vi "delete vi from lib.vi"(8 "error in":errorcluster, 9 "delete on disk (t)":bool=TRUE, 10 "relative path":string, 11 "Project in":refnum<vi>) -> (0 "error out":errorcluster, 3 "Project out":refnum<vi>, 5 "lib path":path)   [LabVIEW 2013, in "FixedChannelTBModuleDecideFeatures.lvclass"]
uses:
  FixedChannelTBModuleDecideFeatures.lvclass
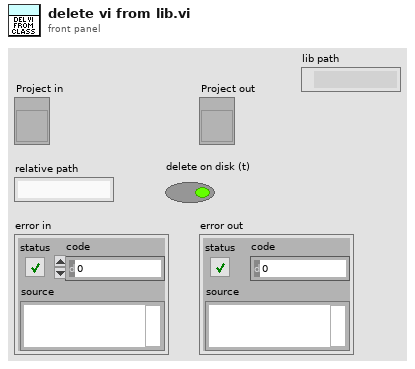
[diagram p1: front panel]
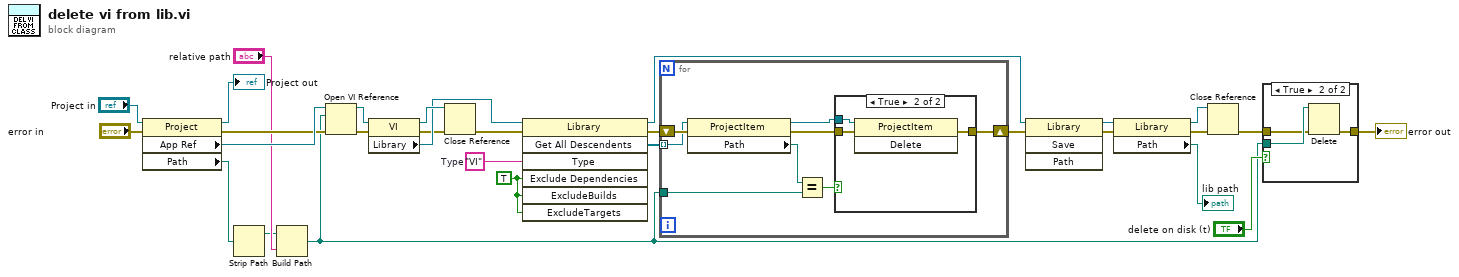
[diagram p0: block diagram]
diagram:
  w18 = TRUE
  w19 = "VI"  # Type
  n1 = property class="Project"(reference="Project in", error in="error in") -> (reference out=→"Project out":refnum<vi>, error out=w14:errorcluster, "App Ref"=w15:refnum<vi>, "Path"=w11:path)
  n2 = Strip Path(path=w11) -> (stripped path=w12:path)  [unwired: 1 out]
  n3 = Build Path(base path=w12, name or relative path="relative path") -> (appended path=w7:path)
  n4 = Open VI Reference(application reference (local)=w15, vi path=w7, error in (no error)=w14) -> (vi reference=w16:refnum<vi>, error out=w17:errorcluster)  [unwired: 3 in]
  n5 = property class="VI"(reference=w16, error in=w17) -> (reference out=w28:refnum<vi>, error out=w20:errorcluster, "Library"=w21:refnum<vi>)
  n6 = Close Reference(reference=w28, error in (no error)=w20) -> (error out=w27:errorcluster)
  n7 = invoke class="Library" method="Get All Descendents"(reference=w21, error in=w27, "Type"=w19, "Exclude Dependencies"=w18, "ExcludeBuilds"=w18, "ExcludeTargets"=w18) -> (reference out=w26:refnum<vi>, error out=w23:errorcluster, "All Descendents"=w22:refnum<vi>[])  [unwired: 1 in, 4 out]
  n8 = for {
    tunnel: w22 -> [w36] mode=indexing
    shift-right: [w30] -> w24
    shift-left: w23 -> [w37]
    tunnel: w7 -> [w34]
    n9 = property class="ProjectItem"(reference=w36, error in=w37) -> (reference out=w31:refnum<vi>, error out=w32:errorcluster, "Path"=w35:path)
    n10 = Equal?(x=w35, y=w34) -> (x = y?=w33:bool)
    n11 = case shown="True" w33 {
      tunnel: w32 -> [w38 w40]
      tunnel: w31 -> [_ w41]
      tunnel: [w38 w39] -> w30
      frame False {
      }
      frame True {
        n12 = invoke class="ProjectItem" method="Delete"(reference=w41, error in=w40) -> (error out=w39:errorcluster)  [unwired: 1 in, 2 out]
      }
    }
  }
  n13 = invoke class="Library" method="Save"(reference=w26, error in=w24) -> (reference out=w3:refnum<vi>, error out=w25:errorcluster)  [unwired: 2 in, 2 out]
  n14 = property class="Library"(reference=w3, error in=w25) -> (reference out=w2:refnum<vi>, error out=w4:errorcluster, "Path"=→"lib path":path)
  n15 = Close Reference(reference=w2, error in (no error)=w4) -> (error out=w6:errorcluster)
  n16 = case shown="True" "delete on disk (t)" {
    tunnel: w7 -> [_ w45]
    tunnel: w6 -> [w42 w44]
    tunnel: [w42 w43] -> w5
    frame False {
    }
    frame True {
      n17 = Delete(path (use dialog)=w45, error in=w44) -> (error out=w43:errorcluster)  [unwired: 3 in, 2 out]
    }
  }
  "error out" <- w5
